vi "Write Tag Tree.vi"(10 "Tag Tree Out":refnum<class "Tag Tree.lvclass">, 11 "Process Tree View in":refnum<class "Process Tree View.lvclass">) -> (3 "Process Tree View out":refnum<class "Process Tree View.lvclass">)   [LabVIEW 2020, in "Process Tree View.lvclass"]
uses:
  Process Tree View.lvclass
  Tree Helpers/Tag Tree/Tag Tree.lvclass
  Process Tree View.lvclass/Process Tree View.ctl
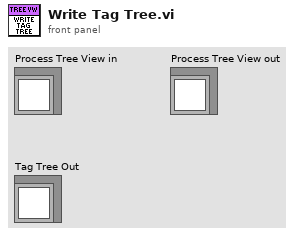
[diagram p1: front panel]
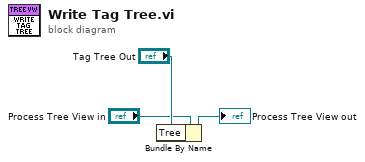
[diagram p0: block diagram]
diagram:
  n1 = Bundle By Name(cluster="Process Tree View in", "Tree"="Tag Tree Out") -> (→"Process Tree View out":refnum<class "Process Tree View.lvclass">)
